vi "ZLIB Path to Path String__ogtk.vi"(4 "error in (no error)":errorcluster, 7 "LV file path":path) -> (0 "error in (no error)":errorcluster, 3 "path string":string)   [LabVIEW 2019]
doc: "Converts a LabVIEW path into a platform specific path string. Almost the same\nas the LabVIEW Path To String function but converts on MacOSX from the HFS\npath syntax into a posix path."
uses:
  <userlib>/_OpenG.lib/lvzip/lvzlib.dll
panel:
  # "Please visit http://www.OpenG.org to learn about the\nOpen Source LabVIEW software movement.\n\nNOTICE -- YOU MUST LEAVE THIS NOTICE IN PLACE.  PER THE TERMS OF THE LICENSE BELOW, YOU MAY SUBLICENSE THIS SOFTWARE \nIN ANY WAY THAT DOES NOT CONFLICT WITH THIS LICENSE.\n\n### BSD License (http://www.opensource.org/licenses/bsd-license.php) Begin ###\n \nCopyright (C) 2006 Rolf Kalbermatter rolf.kalbermatter@citeng.com\nCopyright (C) 2003-2004 Jim Kring jim@jimkring.com\n\nAll rights reserved.\n\nRedistribution and use in source and binary forms, with or without modification, are permitted provided that the following conditions are met:\n\n    * Redistributions of source code must retain the above copyright notice, this list of conditions and the following disclaimer.\n    * Redistributions in binary form must reproduce the above copyright notice, this list of conditions and the following disclaimer in the \n       documentation and/or other materials provided with the distribution.\n    * Neither the name of SciWare, James Kring, Inc., nor the names of its contributors may be used to endorse or promote products derived \n       from this software without specific prior written permission.\n\nTHIS SOFTWARE IS PROVIDED BY THE COPYRIGHT HOLDERS AND CONTRIBUTORS \"AS IS\" AND ANY EXPRESS OR IMPLIED WARRANTIES, \nINCLUDING, BUT NOT LIMITED TO, THE IMPLIED WARRANTIES OF MERCHANTABILITY AND FITNESS FOR A PARTICULAR PURPOSE ARE \nDISCLAIMED. IN NO EVENT SHALL THE COPYRIGHT OWNER OR CONTRIBUTORS BE LIABLE FOR ANY DIRECT, INDIRECT, INCIDENTAL,\n SPECIAL, EXEMPLARY, OR CONSEQUENTIAL DAMAGES (INCLUDING, BUT NOT LIMITED TO, PROCUREMENT OF SUBSTITUTE GOODS OR \nSERVICES; LOSS OF USE, DATA, OR PROFITS; OR BUSINESS INTERRUPTION) HOWEVER CAUSED AND ON ANY THEORY OF LIABILITY, \nWHETHER IN CONTRACT, STRICT LIABILITY, OR TORT (INCLUDING NEGLIGENCE OR OTHERWISE) ARISING IN ANY WAY OUT OF THE USE \nOF THIS SOFTWARE, EVEN IF ADVISED OF THE POSSIBILITY OF SUCH DAMAGE.\n\n### BSD License End ###"
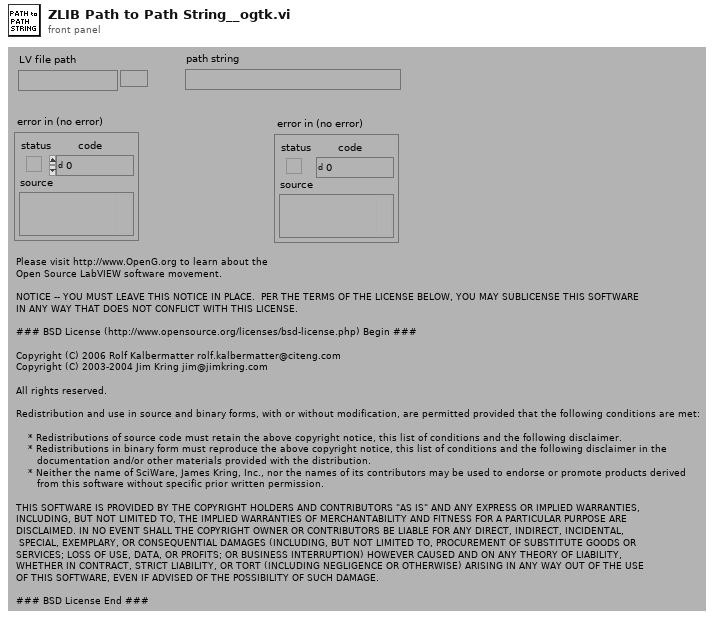
[diagram p1: front panel]
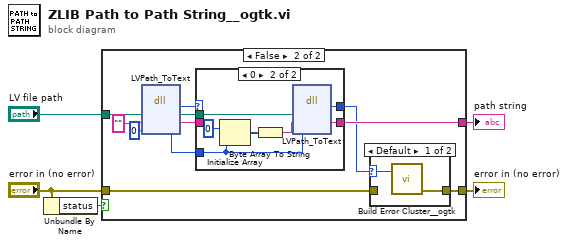
[diagram p0: block diagram]
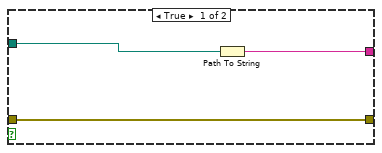
[diagram p2: hidden frame]
diagram:
  n1 = Unbundle By Name("error in (no error)") -> ("status"=w1:bool)
  n2 = case shown="False" w1 {
    tunnel: "LV file path" -> [w8 w19]
    tunnel: [w7 w12] -> w4
    tunnel: [w6 w11] -> w3
    tunnel: "error in (no error)" -> [w6 w9]
    frame True {
      n3 = Path To String(path=w8) -> (string=w7:string)
    }
    frame False {
      n4 = dll-call lib="C:/Program Files (x86)/National Instruments/LabVIEW 2020/user.lib/_OpenG.lib/lvzip/lvzlib.*" fn="LVPath_ToText"("LV file path"=w19, "string"="", "len"=0) -> (w18:i32, "LV file path"=w17:path, "string"=w13:string, "len"=w14:i32)  [unwired: 3 in, 2 out]
      n5 = case shown="0" w18 {
        selector: w18 -> [w24 _]
        tunnel: w17 -> [_ w31]
        tunnel: [w24 w30] -> w10
        tunnel: w14 -> [_ w28]
        tunnel: w13 -> [w23 _]
        tunnel: [w23 w25] -> w12
        frame Default {
        }
        frame 0 {
          n6 = Initialize Array(u8 0 ("Element Data"), w28) -> (w27:u8[])
          n7 = Byte Array To String(unsigned byte array=w27) -> (string=w26:string)
          n8 = dll-call lib="C:/Program Files (x86)/National Instruments/LabVIEW 2020/user.lib/_OpenG.lib/lvzip/lvzlib.*" fn="LVPath_ToText"("LV file path"=w31, "string"=w26, "len"=w28) -> (w30:i32, "string"=w25:string)  [unwired: 5 in, 2 out]
        }
      }
      n9 = case shown="Default" w10 {
        selector: w10 -> [w20 _]
        tunnel: w9 -> [_ w22]
        tunnel: [w21 w22] -> w11
        frame Default {
          n10 = call "Build Error Cluster__ogtk.vi"("code"=w20) -> ("error out"=w21:errorcluster)  [unwired: 1 in]
        }
        frame 0 {
        }
      }
    }
  }
  "path string" <- w4
  "error in (no error)" <- w3
